vi "List Entries.vi"(0 "BroadcastRegistry in":refnum<class "BroadcastRegistry.lvclass">) -> (4 "BroadcastRegistry out":refnum<class "BroadcastRegistry.lvclass">, 6 "Array":string[](array[string]))   [LabVIEW 2020, in "Communicable State Machine.lvlib" / "BroadcastRegistry.lvclass"]
uses:
  BroadcastRegistry.lvclass
  BroadcastRegistry.lvclass/BroadcastRegistry.ctl
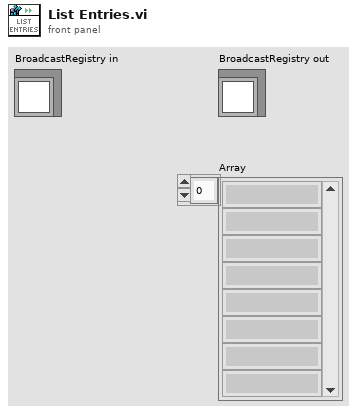
[diagram p1: front panel]
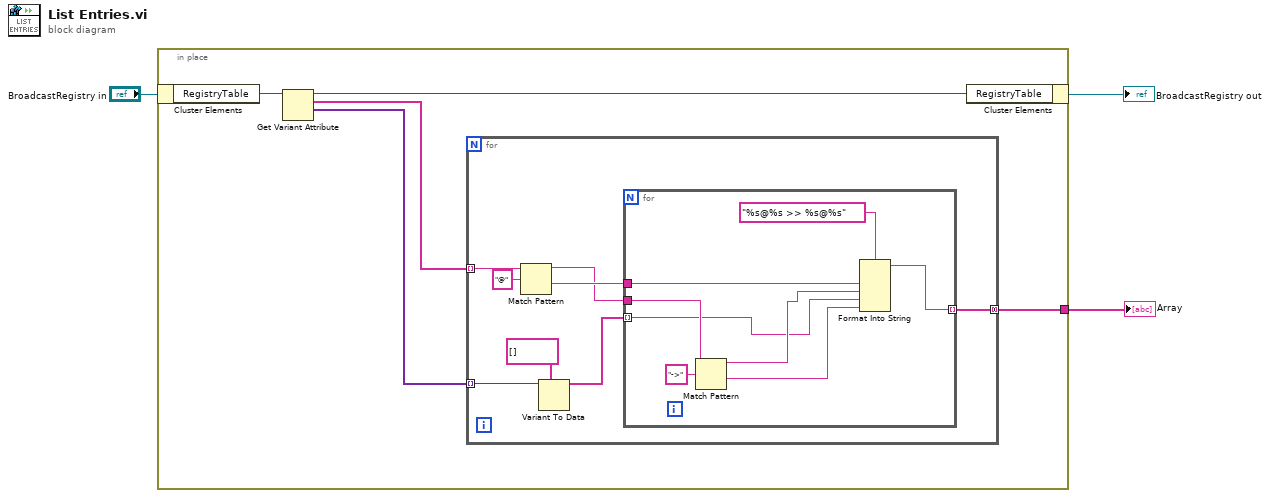
[diagram p0: block diagram]
diagram:
  n1 = in-place {
    in-place-border: [w4] -> w1
    n2 = in-place-cluster #1("BroadcastRegistry in") -> ("RegistryTable"=w8:variant)
    n3 = Get Variant Attribute(Variant=w8) -> (duplicate Variant=w7:variant, names=w5:string[], values=w6:variant[])  [unwired: 3 in, 1 out]
    n4 = for {
      tunnel: w6 -> [w16] mode=indexing
      tunnel: w5 -> [w14] mode=indexing
      tunnel: [w9] -> w4 mode=concatenating
      n5 = Match Pattern(string=w14, regular expression="@") -> (before substring=w11:string, after substring=w12:string)  [unwired: 1 in, 2 out]
      n6 = Variant To Data(type=string[] [], Variant=w16) -> (data=w10:string[])  [unwired: 1 in, 1 out]
      n7 = for {
        tunnel: w12 -> [w21]
        tunnel: w11 -> [w24]
        tunnel: w10 -> [w19] mode=indexing
        tunnel: [w17] -> w9 mode=indexing
        n8 = Match Pattern(string=w24, regular expression="->") -> (before substring=w20:string, after substring=w18:string)  [unwired: 1 in, 2 out]
        n9 = Format Into String(format string="%s@%s >> %s@%s", w21, w20, w19, w18) -> (resulting string=w17:string)  [unwired: 2 in, 1 out]
      }
    }
    n10 = in-place-cluster #1("RegistryTable"=w7) -> (→"BroadcastRegistry out":refnum<class "BroadcastRegistry.lvclass">)
  }
  "Array" <- w1
